vi "Set Wet Air Flow Rate.vi"(8 "error in":errorcluster, 10 "Wet Air Flow Rate (ml/min)":i32, 11 "OVG In":refnum<class "Owlstone GEN-SYS.lvclass">) -> (0 "error out":errorcluster, 3 "OVG Out":refnum<class "Owlstone GEN-SYS.lvclass">)   [LabVIEW 2011, in "Owlstone GEN-SYS.lvclass"]
uses:
  Owlstone GEN-SYS.lvclass
  Owlstone GEN-SYS.lvclass/Owlstone GEN-SYS.ctl
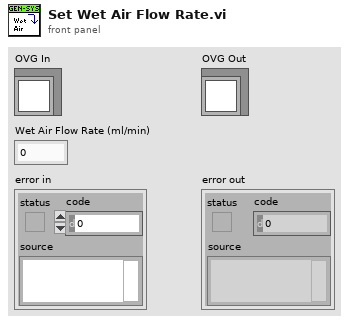
[diagram p1: front panel]
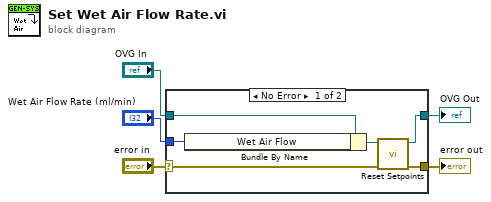
[diagram p0: block diagram]
diagram:
  n1 = case shown="No Error" "error in" {
    selector: "error in" -> [w9 w13]
    tunnel: "Wet Air Flow Rate (ml/min)" -> [w6 _]
    tunnel: [w8 w13] -> w3
    tunnel: "OVG In" -> [w11 w12]
    tunnel: [w7 w12] -> w1
    frame No Error {
      n2 = Bundle By Name(cluster=w11, "Wet Air Flow"=w6) -> (w10:refnum<class "Owlstone GEN-SYS.lvclass">)
      n3 = call "Reset Setpoints.vi"("error in (no error)"=w9, "Owlstone GEN-SYS in"=w10) -> ("error out"=w8:errorcluster, "Owlstone GEN-SYS out"=w7:refnum<class "Owlstone GEN-SYS.lvclass">)  [unwired: 8 in]
    }
    frame Error {
    }
  }
  "error out" <- w3
  "OVG Out" <- w1
